vi "GT_SetJogPrm.vi"(3 "pPrm":cluster{"acc":dbl, "dec":dbl, "smooth":dbl}, 4 "Axis in":T1=1 items=["Axis Control"=0, "Axis 1"=1, "Axis 2"=2, "Axis 3"=3, "Axis 4"=4, "Axis 5"=5, "Axis 6"=6, "Axis 7"=7, "Axis 8"=8, "Vector Space Control"=16, "Vector Space 1"=17, "Vector Space 2"=18, "Vector Space 3"=19, "Vector Space 4"=20], 5 "rtn_In":cluster{"rtn":i16, "Func":string}) -> (0 "pPrm":cluster{"acc":dbl, "dec":dbl, "smooth":dbl}, 1 "Axis out":T1=1 items=["Axis Control"=0, "Axis 1"=1, "Axis 2"=2, "Axis 3"=3, "Axis 4"=4, "Axis 5"=5, "Axis 6"=6, "Axis 7"=7, "Axis 8"=8, "Vector Space Control"=16, "Vector Space 1"=17, "Vector Space 2"=18, "Vector Space 3"=19, "Vector Space 4"=20], 2 "rtn_Out":cluster{"rtn":i16, "Func":string})   [LabVIEW 2014]
uses:
  <vilib>/Motion/FlexMotion/CustomControls/CustomControls.llb/AxisOrVectorSpaceControl To Control.flx
  VC6/gts.dll
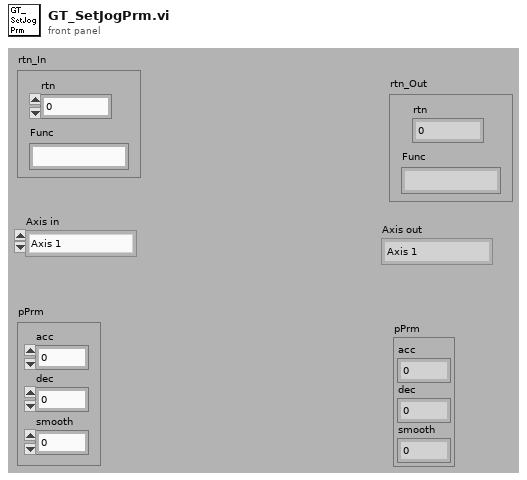
[diagram p1: front panel]
types:
  T1 = typedef "AxisOrVectorSpaceControl To Control.flx" = u16
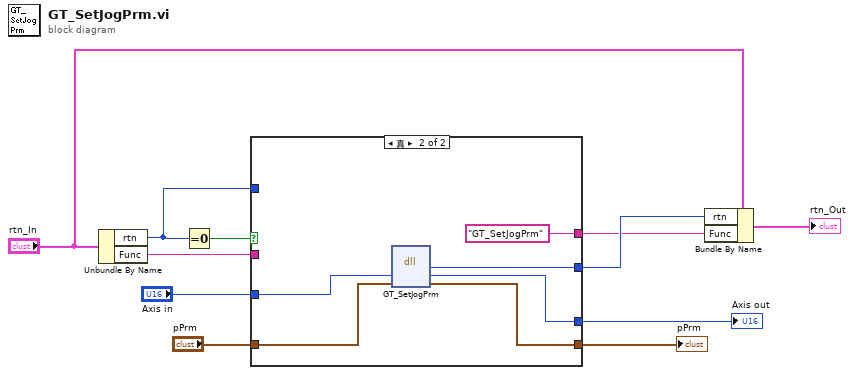
[diagram p0: block diagram]
diagram:
  n1 = Unbundle By Name("rtn_In") -> ("rtn"=w2:i16, "Func"=w1:string)
  n2 = Equal To 0?(x=w2) -> (x = 0?=w11:bool)
  n3 = case shown="真" w11 {
    tunnel: "Axis in" -> [w13 w21]
    tunnel: [w13 w20] -> w9
    tunnel: [w15 w19] -> w6
    tunnel: [w14 "GT_SetJogPrm" ("Func")] -> w5
    tunnel: "pPrm" -> [w12 w17]
    tunnel: [w12 w16] -> w3
    tunnel: w2 -> [w15 _]
    tunnel: w1 -> [w14 _]
    frame False {
    }
    frame True {
      n4 = dll-call lib="PTH2Fabs DNewGTS AC-800LWin7版源程序-20170926gts85VC6gts.dll" fn="GT_SetJogPrm"("proFile"=w21, "pPrm"=w17) -> ("rtn"=w19:i16, "proFile"=w20:i16, "pPrm"=w16:cluster{"acc":dbl, "dec":dbl, "smooth":dbl})  [unwired: 3 in, 2 out]
    }
  }
  "Axis out" <- w9
  "pPrm" <- w3
  n5 = Bundle By Name(cluster="rtn_In", "rtn"=w6, "Func"=w5) -> (→"rtn_Out":cluster{"rtn":i16, "Func":string})
